vi "sleep_deprivation_mode.vi"(8 "Input \nparameters":T2={"Frame rate (ms)"=2000, "Worm strain"="N2", "# Images"=0, "State"=enum."Image acquisition", "Time elapsed"=0.0, "Max_num_runs"=100000, "#TTL"=0, "Time of start TTL"=100000, "ImSub Value"=0, "Time of last TTL"=0, "Number of Columns"=2, "Number of Rows"=2, "# AdjacentTTL"=0, "Sleep deprivation status"="", "Sleep Detection"=FALSE, "# Sleep detections"=0, "Time of first sleep detection"=0, "Time max # adjacent TTL"=0, "Image t-1"=[], "Image t"=[]} {"Number of Rows" items=["1"=1, "2"=2, "3"=3, "4"=4]; "Number of Columns" items=["1"=1, "2"=2, "3"=3, "4"=4]}, 9 "#TTL change\nmode":dbl=10000.0, 10 "Second \nDeprivation Method":T3={"lines"="Dev1/port2/line7", "Pause time (ms)"=0, "Pulse length (ms)"=300, "# Pulses"=1}, 11 "First \nDeprivation Method":T3={"lines"="Dev1/port2/line6", "Pause time (ms)"=0, "Pulse length (ms)"=15, "# Pulses"=1}) -> ()   [LabVIEW 2011]
uses:
  state.ctl
panel:
  # "Line 6 Tap Magnet"
  # "Line 7 LED"
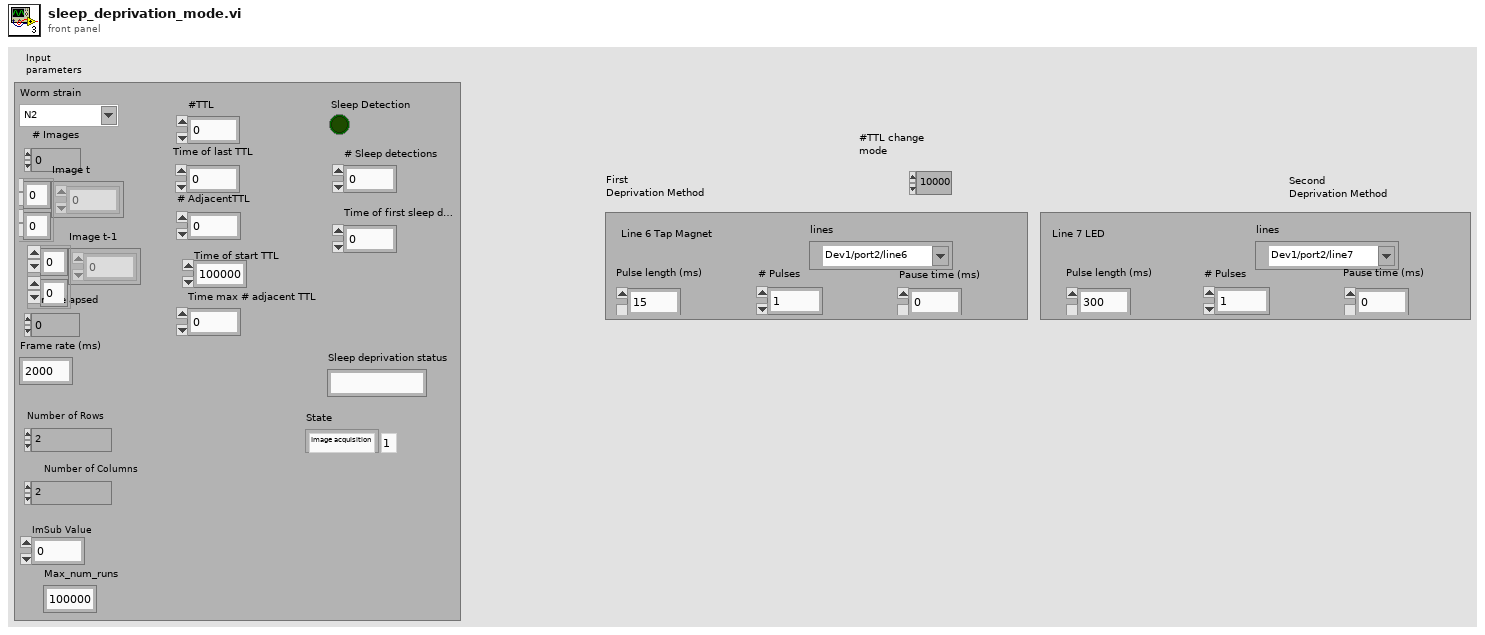
[diagram p1: front panel]
types:
  T1 = typedef "state.ctl" = enum16{"Initialize measurement", "Image acquisition", "Image processing", "Sleep detection", "Control TTL protocol ", "Sleep deprivation", "Update image & exit condition", "Wait "}
  T2 = cluster{"Frame rate (ms)":u32, "Worm strain":string, "# Images":i32, "State":T1, "Time elapsed":dbl, "Max_num_runs":i32, "#TTL":i32, "Time of start TTL":i32, "ImSub Value":i32, "Time of last TTL":i32, "Number of Columns":u32, "Number of Rows":u32, "# AdjacentTTL":i32, "Sleep deprivation status":string, "Sleep Detection":bool, "# Sleep detections":i32, "Time of first sleep detection":i32, "Time max # adjacent TTL":i32, "Image t-1":i32[][], "Image t":i32[][]}
  T3 = cluster{"lines":tag, "Pause time (ms)":u32, "Pulse length (ms)":u32, "# Pulses":i32}
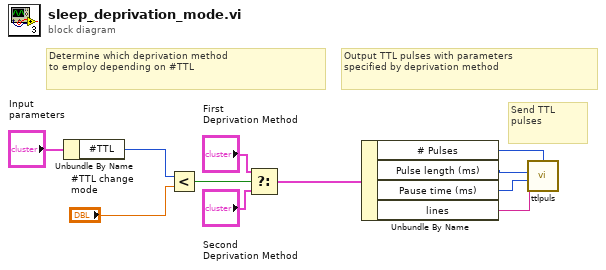
[diagram p0: block diagram]
diagram:
  # "Send TTL \npulses"
  # "Output TTL pulses with parameters\nspecified by deprivation method"
  # "Determine which deprivation method\nto employ depending on #TTL"
  n1 = Unbundle By Name("Input \nparameters") -> ("#TTL"=w11:i32)
  n2 = Less?(x=w11, y="#TTL change\nmode") -> (x < y?=w2:bool)
  n3 = Select(t="First \nDeprivation Method", s=w2, f="Second \nDeprivation Method") -> (s? t:f=w4:T3)
  n4 = Unbundle By Name(w4) -> ("# Pulses"=w8:i32, "Pulse length (ms)"=w7:u32, "Pause time (ms)"=w6:u32, "lines"=w5:tag)
  n5 = call "ttlpuls.vi"("lines"=w5, "Pause Time (ms)"=w6, "Pulse Length (ms)"=w7, "Number of Pulses"=w8) -> ()
